vi "Set Output Values.vi"(6 "Fundamental Frequency (0.0 Hz)":dbl min=0.0 max=1200000.0 format="%^.3e", 7 "Output Value(s) (0 - Amplitude)":u32(ring) items=["Amplitude", "Volts dc or update volts ac", "Volts ac dBm update", "Volts ac or volts dc with 0 Hz", "Volts ac in dBm", "Current dc or update current ac", "Current ac", "Update frequency", "Resistance", "Capacitance", "Temperature (Celsius)", "Temperature (Fahrenheit)", "Power dc or update power ac", "Power ac", "Dual volts dc or update dual ac", "Dual volts ac in volts", "Power ac in dBm update", "Power ac in dBm", "Dual volts ac in dBm update", "Dual volts ac in dBm"], 8 "error in (no error)":errorcluster, 9 "Secondary Value (0.0)":dbl format="%^.3e", 10 "Primary Value (0.0)":dbl format="%^.3e", 11 "VISA resource name":refnum<visa-resource-name>) -> (0 "error out":errorcluster {"code" format="%.0x"}, 3 "VISA resource name out":refnum<visa-resource-name>)   [LabVIEW 2016, in "Fluke 5XXX Series Multicalibrators.lvlib"]
doc: "This VI sets the output of the Calibrator and establishes a new reference point for the error mode. If only one amplitude is supplied, the Calibrator sources a single output. If two amplitudes are supplied, the Calibrator sources two outputs. The second amplitude will be sourced at the AUX terminals for dual voltage outputs. If the frequency is not supplied, the Calibrator will use the frequency that is presently in use.\n\nNotes:\n\n(1) Instrument models 5700A, 5720A and 57LFC are not equipped with dual outpus. Only single output operations are available.\n\n(2) To source or measure a temperature, select the desired sensor and sensor parameters first (instrument models 5500A and 5520A only).\n\n(3) To source a signal using the Calibrator scope options, refer to the Oscilloscope Functions (instrument models 5500A and 5520A only).\n\n(4) If you change the frequency of an ac function and the harmonic output is not explicitly set at the same time with the function Set Harmonic, the harmonic will be set to 1 (instrument models 5500A and 5520A only)."
uses:
  Fluke 5XXX Series Multicalibrators.lvlib
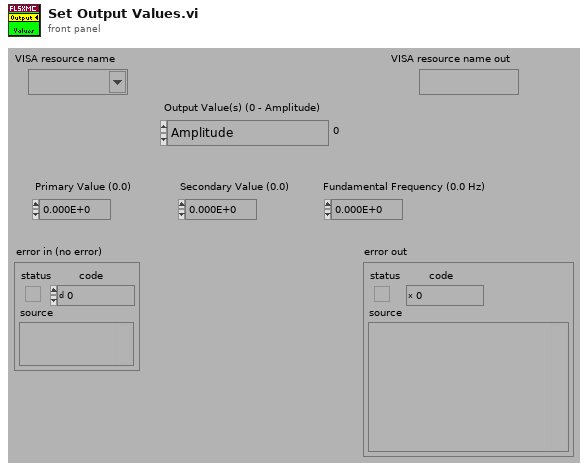
[diagram p1: front panel]
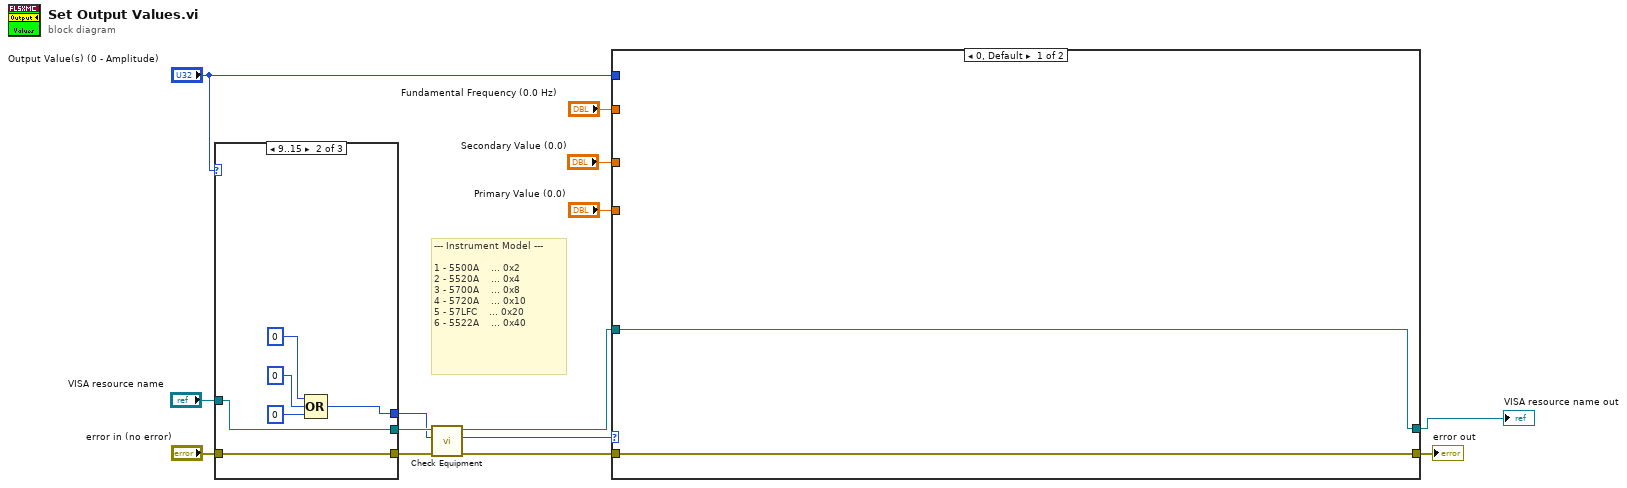
[diagram p0: block diagram]
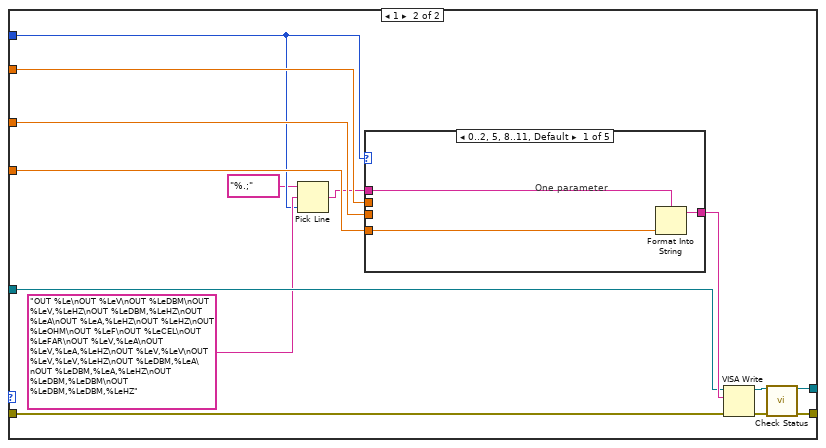
[diagram p2: hidden frame]
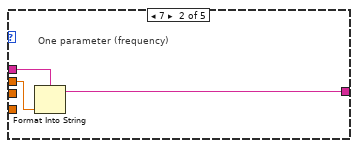
[diagram p3: hidden frame]
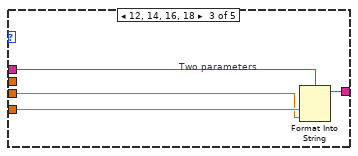
[diagram p4: hidden frame]
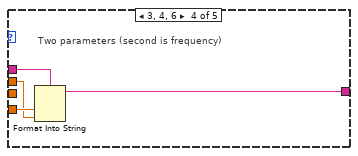
[diagram p5: hidden frame]
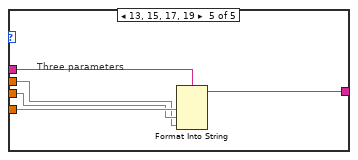
[diagram p6: hidden frame]
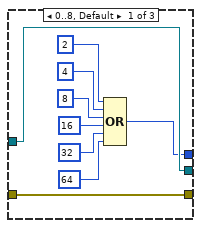
[diagram p7: hidden frame]
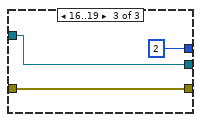
[diagram p8: hidden frame]
diagram:
  # "--- Instrument Model ---\n\n1 - 5500A    ... 0x2\n2 - 5520A    ... 0x4\n3 - 5700A    ... 0x8\n4 - 5720A    ... 0x10\n5 - 57LFC    ... 0x20\n6 - 5522A    ... 0x40"
  n1 = case shown="9..15" "Output Value(s) (0 - Amplitude)" {
    tunnel: "VISA resource name" -> [w18 w27 w31]
    tunnel: "error in (no error)" -> [w19 w25 w30]
    tunnel: [w18 w27 w31] -> w3
    tunnel: [w19 w25 w30] -> w4
    tunnel: [w17 w26 2 ("Numeric")] -> w2
    frame 0..8, Default {
      n2 = Compound Arithmetic op=OR(u32 2 ("Numeric"), u32 4 ("Numeric"), u32 8 ("Numeric"), u32 16 ("Numeric"), u32 32 ("Numeric"), 64 ("Numeric")) -> (w17:u32)
    }
    frame 9..15 {
      n3 = Compound Arithmetic op=OR(0 ("Numeric"), 0 ("Numeric"), 0 ("Numeric")) -> (w26:i32)
    }
    frame 16..19 {
    }
  }
  n4 = call "Check Equipment.vi"("error in (no error)"=w4, "Bit Mask"=w2, "VISA resource name"=w3) -> ("error out"=w5:errorcluster, "Present?"=w1:u32, "VISA resource name out"=w6:refnum<visa-resource-name>)  [unwired: 6 in]
  n5 = case shown="0, Default" w1 {
    tunnel: w6 -> [w34 w46]
    tunnel: w5 -> [w33 w45]
    tunnel: [w34 w41] -> w12
    tunnel: [w33 w39] -> w11
    tunnel: "Output Value(s) (0 - Amplitude)" -> [_ w37]
    tunnel: "Primary Value (0.0)" -> [_ w48]
    tunnel: "Fundamental Frequency (0.0 Hz)" -> [_ w44]
    tunnel: "Secondary Value (0.0)" -> [_ w43]
    frame 0, Default {
    }
    frame 1 {
      n6 = Pick Line(string ("")="%.;", multi-line string="OUT %Le\nOUT %LeV\nOUT %LeDBM\nOUT %LeV,%LeHZ\nOUT %LeDBM,%LeHZ\nOUT %LeA\nOUT %LeA,%LeHZ\nOUT %LeHZ\nOUT %LeOHM\nOUT %LeF\nOUT %LeCEL\nOUT %LeFAR\nOUT %LeV,%LeA\nOUT %LeV,%LeA,%LeHZ\nOUT %LeV,%LeV\nOUT %LeV,%LeV,%LeHZ\nOUT %LeDBM,%LeA\nOUT %LeDBM,%LeA,%LeHZ\nOUT %LeDBM,%LeDBM\nOUT %LeDBM,%LeDBM,%LeHZ", line index=w37) -> (output string=w36:string)
      n7 = case shown="0..2, 5, 8..11, Default" w37 {
        tunnel: w48 -> [w51 _ w58 w62 w67]
        tunnel: [w50 w54 w56 w60 w64] -> w47
        tunnel: w44 -> [_ w53 _ w61 w65]
        tunnel: w43 -> [_ _ w57 _ w66]
        tunnel: w36 -> [w49 w52 w55 w59 w63]
        frame 0..2, 5, 8..11, Default {
          # "One parameter"
          n8 = Format Into String(format string=w49, w51) -> (resulting string=w50:string)  [unwired: 2 in, 1 out]
        }
        frame 7 {
          # "One parameter (frequency)"
          n9 = Format Into String(format string=w52, w53) -> (resulting string=w54:string)  [unwired: 2 in, 1 out]
        }
        frame 12, 14, 16, 18 {
          # "Two parameters"
          n10 = Format Into String(format string=w55, w58, w57) -> (resulting string=w56:string)  [unwired: 2 in, 1 out]
        }
        frame 3, 4, 6 {
          # "Two parameters (second is frequency)"
          n11 = Format Into String(format string=w59, w62, w61) -> (resulting string=w60:string)  [unwired: 2 in, 1 out]
        }
        frame 13, 15, 17, 19 {
          # "Three parameters"
          n12 = Format Into String(format string=w63, w67, w66, w65) -> (resulting string=w64:string)  [unwired: 2 in, 1 out]
        }
      }
      n13 = VISA Write(VISA resource name=w46, write buffer=w47, error in (no error)=w45) -> (VISA resource name out=w42:refnum<visa-resource-name>, error out=w40:errorcluster)  [unwired: 1 out]
      n14 = call "Check Status.vi"("VISA resource name"=w42, "error in (no error)"=w40) -> ("VISA resource name out"=w41:refnum<visa-resource-name>, "error out"=w39:errorcluster)  [unwired: 12 in]
    }
  }
  "VISA resource name out" <- w12
  "error out" <- w11
